vi "OSC_Calc.vi"() -> ()   [LabVIEW 2014]
uses:
  <vilib>/gmath/NI_Gmath.lvlib
panel:
  in  "Lambda 2":dbl=2.0
  in  "Lambda 1":dbl=2.0
  in  "Air MFC Delivery":dbl=2.0
  in  "Test Number":i32
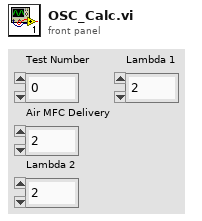
[diagram p1: front panel]
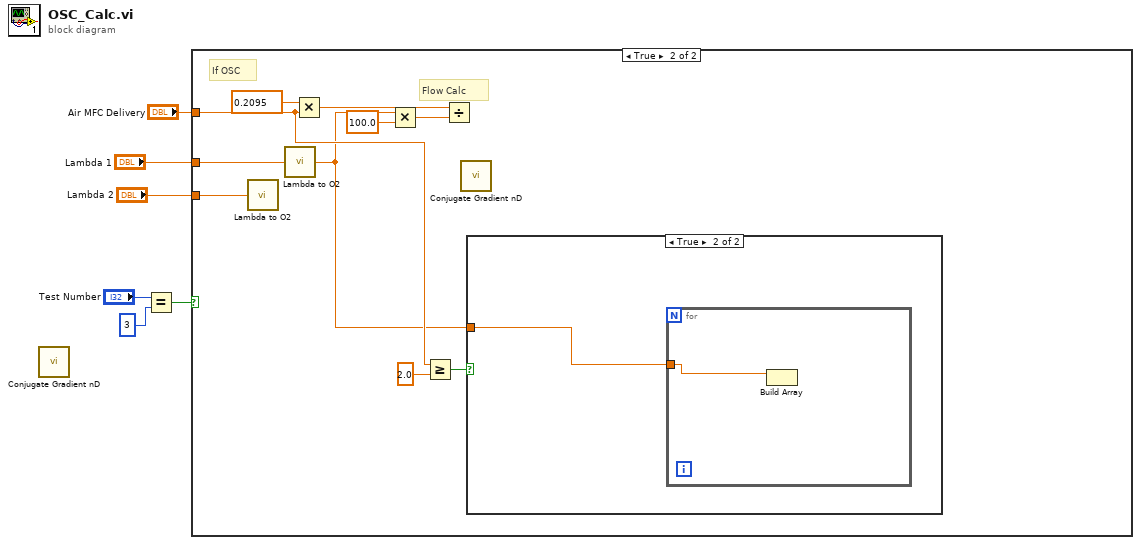
[diagram p0: block diagram]
diagram:
  n1 = call <vilib>:"Conjugate Gradient nD.vi"() -> ()  [unwired: 6 in, 4 out]
  n2 = Equal?(x="Test Number", y=3 ("length")) -> (x = y?=w6:bool)
  n3 = case shown="True" w6 {
    tunnel: "Air MFC Delivery" -> [_ w9]
    tunnel: "Lambda 1" -> [_ w16]
    tunnel: "Lambda 2" -> [_ w15]
    frame False {
    }
    frame True {
      # "Flow Calc"
      # "If OSC"
      n4 = call "Lambda to O2.vi"("Lambda"=w15) -> ()  [unwired: 1 out]
      n5 = call "Lambda to O2.vi"("Lambda"=w16) -> ("O2 %"=w7:sgl)
      n6 = Multiply(x=0.2095, y=w9) -> (x*y=w13:dbl)
      n7 = Multiply(x=w7, y=sgl 100.0) -> (x*y=w12:sgl)
      n8 = Greater Or Equal?(x=w9, y=2.0) -> (x >= y?=w10:bool)
      n9 = Divide(x=w13, y=w12) -> ()  [unwired: 1 out]
      n10 = call <vilib>:"Conjugate Gradient nD.vi"() -> ()  [unwired: 6 in, 4 out]
      n11 = case shown="True" w10 {
        tunnel: w7 -> [_ w17]
        frame False {
        }
        frame True {
          n12 = for {
            tunnel: w17 -> [w18]
            n13 = Build Array(w18) -> ()  [unwired: 1 in, 1 out]
          }
        }
      }
    }
  }
